vi "Digilens DLP Gen2 UI .vi"(11 "TopLevel In":refnum<class "TopLevel.lvclass">) -> (3 "TopLevel Out":refnum<class "TopLevel.lvclass">)   [LabVIEW 2022 SP3, in "TopLevel.lvclass"] (continued)
    shift-left: _ -> [w28]
    shift-right: [w32] -> _
    shift-left: w6 -> [w26]
    shift-right: [w31] -> _
    shift-left: w16 -> [w33]
    tunnel: w5 -> [w25]
    tunnel: [w24] -> w14
    shift-right: [w23] -> _
    shift-left: _ -> [w22]
    tunnel: w7 -> [_]
    tunnel: w1 -> [w21]
    tunnel: w2 -> [w20]
    stop <- w30 stop-if-true
    w27 = -1  # Timeout
    n10 = call <vilib>:"Parse State Queue__JKI_lib_State_Machine.vi"("State Queue"=w33, "Error In (no error)"=w26) -> ("Remaining States"=w35:string, "Current State"=w36:string, "Arguments"=w34:string)  [unwired: 11 in]
    n11 = case shown="\"Action: Apply Process Mode\"" w36 {
      selector: w36 -> [_ _ w2966 _ _ _ _ _ _ _ _ _ _ _ _ _ _ _ _ _ _ _ _ _ _ _ _ _ _ _ _ _ _ _ _ _ _ _ _ _ _ _ _ _ _ _ _ _ _ _ _ _ _ _ _ _ _ _ _ _ _ _ _ _ _ _ _ _ _ _ _ _ _ _ _ _ _ _ _ _ _ _ _ _ _ _ _ _ _]
      tunnel: w35 -> [w46 w2963 w2970 w2990 w2998 w3005 w3011 w3023 w3036 w3056 w3067 w3078 w3098 w3123 w3140 w3152 w3158 w3206 w3325 w3339 w3351 w3357 w3365 w3373 w3388 w3428 w3519 w3605 w3616 w3626 w3637 w3662 w3706 w3716 w3750 w3756 w3780 w3793 w3891 w3913 w3934 w3947 w3984 w4007 w4014 w4021 w4040 w4045 w4079 w4087 w4092 w4106 w4108 w4119 w4140 w4145 w4154 w4164 w4168 w4181 w4185 w4193 w4238 w4249 w4282 w4309 w4360 w4405 w4409 w4438 w4514 w4521 w4528 w4530 w4567 w4619 w4660 w4689 w4693 w4703 w4707 w4710 w4726 w4730 w4775 w4819 w4824 w4839 w4863]
      tunnel: w34 -> [_ _ _ _ _ _ _ _ _ _ _ _ w3086 w3109 w3130 w3148 _ _ _ _ _ _ w3358 _ _ _ w3513 _ _ _ _ _ _ _ _ _ _ _ _ w3905 w3929 w3942 _ _ _ _ _ _ _ _ _ _ _ _ _ _ _ _ _ _ _ w4190 _ w4248 _ _ _ _ _ w4430 _ _ _ _ _ _ _ _ _ _ _ _ _ w4728 w4768 _ _ w4833 w4859]
      tunnel: w28 -> [w44 w2960 w2968 w2981 w2995 w3003 w3008 w3019 w3034 w3053 w3063 w3072 w3084 w3115 w3129 w3142 w3153 w3202 _ w3338 w3346 w3354 w3362 w3370 w3383 w3441 w3516 w3600 w3612 w3621 w3634 w3658 w3701 w3711 w3745 w3751 w3775 w3790 w3888 w3908 w3932 w3944 w3981 w4004 w4011 w4018 w4028 w4043 w4075 w4086 w4090 w4094 w4112 w4117 w4139 w4144 w4151 w4161 w4167 w4179 w4184 w4189 w4241 w4245 w4278 w4296 w4348 w4399 w4408 w4445 w4511 w4518 w4525 w4557 w4582 w4622 w4657 w4681 w4692 w4700 w4706 w4716 w4725 w4732 w4777 w4818 w4823 w4834 w4860]
      tunnel: [w43 w2961 w2972 w2987 errorcluster {"status"=FALSE, "code"=0, "source"=""} ("error out") w3002 w3009 w3012 w3025 w3054 w3061 w3070 w3088 w3111 w3126 w3144 w3156 w3200 w3265 w3329 w3347 w3355 w3363 w3371 w3386 w3422 w3517 w3603 w3610 w3624 w3635 w3654 w3704 w3714 w3748 w3754 w3778 w3783 w3836 w3911 w3930 w3939 w3977 w4008 w4012 w4019 w4027 w4044 w4058 w4083 w4091 w4093 w4109 w4114 w4141 w4146 w4148 w4159 w4169 w4176 w4186 w4188 w4234 w4251 w4262 w4299 w4350 w4398 w4410 w4441 w4496 w4516 w4522 w4532 w4572 w4615 w4630 w4685 w4694 w4696 w4708 w4715 w4727 w4735 w4780 w4820 w4825 w4835 w4851] -> w32
      tunnel: w26 -> [w42 w2961 w2971 w2987 w2994 w3002 w3009 w3017 w3024 w3054 w3060 w3069 w3087 w3110 w3125 w3143 w3156 w3199 w3307 w3333 w3348 w3355 w3363 w3371 w3386 w3417 w3517 w3603 w3609 w3624 w3635 w3653 w3704 w3714 w3748 w3754 w3778 w3782 w3836 w3911 w3931 w3945 w3971 w4008 w4012 w4019 w4026 w4044 w4048 w4082 w4091 w4096 w4109 w4113 w4141 w4146 w4147 w4158 w4169 w4175 w4186 w4187 w4244 w4253 w4261 w4295 w4347 w4397 w4410 w4440 w4508 w4515 w4523 w4544 w4579 w4621 w4646 w4684 w4694 w4695 w4708 w4714 w4727 w4734 w4779 w4820 w4825 w4828 w4856]
      tunnel: [w45 w2962 w2969 w2989 w2997 w3004 w3010 w3022 w3035 w3055 w3066 w3078 w3097 w3122 w3139 w3151 w3157 w3205 w3324 w3339 w3350 w3356 w3364 w3372 w3387 w3427 w3518 w3604 w3615 w3625 w3636 w3661 w3705 w3715 w3749 w3755 w3779 w3793 w3891 w3912 w3933 w3946 w3984 w4007 w4013 w4020 w4039 w4045 w4079 w4087 w4092 w4106 w4108 w4119 w4140 w4145 w4154 w4164 w4168 w4181 w4185 w4193 w4239 w4250 w4282 w4309 w4360 w4405 w4409 w4439 w4514 w4521 w4528 w4531 w4568 w4620 w4660 w4689 w4693 w4703 w4707 w4711 w4726 w4731 w4776 w4819 w4824 w4839 w4863] -> w31
      tunnel: [_ _ _ _ _ TRUE _ _ _ _ _ _ _ _ _ _ _ _ _ _ _ _ _ _ _ _ _ _ _ _ _ _ _ _ _ _ _ _ _ _ _ _ _ _ _ _ _ _ _ _ _ _ _ _ _ _ _ _ _ _ _ _ _ _ _ _ _ _ _ _ _ _ _ _ _ _ _ _ _ _ _ _ _ _ _ _ _ _ _] -> w30
      tunnel: [w41 w2960 w2968 w2988 w2995 w3003 w3008 w3016 w3034 w3050 w3059 w3072 w3085 w3115 w3129 w3142 w3153 w3198 w3323 w3332 w3346 w3354 w3362 w3370 w3383 w3432 w3516 w3600 w3612 w3621 w3634 w3658 w3701 w3711 w3745 w3751 w3775 w3789 w3888 w3908 w3932 w3944 w3981 w4004 w4011 w4018 w4028 w4043 w4075 w4086 w4090 w4094 w4112 w4117 w4139 w4144 w4151 w4161 w4167 w4179 w4184 w4189 w4241 w4246 w4278 w4296 w4348 w4399 w4408 w4445 w4509 w4518 w4525 w4538 w4582 w4617 w4638 w4681 w4692 w4700 w4706 w4713 w4725 w4733 w4778 w4818 w4823 w4834 w4860] -> w29
      tunnel: w27 -> [w40 _ _ _ _ _ _ _ _ _ _ _ _ _ _ _ _ _ _ _ _ _ _ _ _ _ _ _ _ _ _ _ _ _ _ _ _ _ _ _ _ _ _ _ _ _ _ _ _ _ _ _ _ _ _ _ _ _ _ _ _ _ _ _ _ _ _ _ _ _ _ _ _ _ _ _ _ _ _ _ _ _ _ _ _ _ _ _ _]
      tunnel: w25 -> [w39 w2959 w2965 w2978 w2992 w3000 w3007 w3021 w3033 w3052 w3065 w3077 w3096 w3121 w3138 w3150 w3155 w3204 w3321 w3337 w3345 w3353 w3361 w3369 w3384 w3446 w3515 w3602 w3614 w3623 w3633 w3660 w3703 w3713 w3747 w3753 w3777 w3792 w3890 w3910 w3928 w3941 w3983 w4006 w4010 w4016 w4031 w4042 w4078 w4085 w4089 w4097 w4111 w4121 w4138 w4143 w4153 w4163 w4166 w4177 w4183 w4192 w4243 w4255 w4281 w4308 w4359 w4404 w4407 w4449 w4513 w4520 w4527 w4559 w4591 w4624 w4659 w4686 w4691 w4702 w4705 w4722 w4724 w4743 w4788 w4817 w4822 w4838 w4862]
      tunnel: [w38 w2959 w2965 w2978 w2992 w3000 w3007 w3021 w3033 w3052 w3065 w3077 w3096 w3121 w3138 w3150 w3155 w3204 w3321 w3337 w3345 w3353 w3361 w3369 w3384 w3446 w3515 w3602 w3614 w3623 w3633 w3660 w3703 w3713 w3747 w3753 w3777 w3792 w3890 w3910 w3928 w3941 w3983 w4006 w4010 w4016 w4031 w4042 w4078 w4085 w4089 w4097 w4111 w4121 w4138 w4143 w4153 w4163 w4166 w4178 w4183 w4192 w4243 w4255 w4281 w4308 w4359 w4404 w4407 w4449 w4513 w4520 w4527 w4559 w4591 w4624 w4659 w4687 w4691 w4702 w4705 w4722 w4724 w4743 w4788 w4817 w4822 w4838 w4862] -> w24
      tunnel: [w37 w2958 w2964 w2977 w2991 w2999 w3006 w3020 w3032 w3051 w3064 w3076 w3095 w3120 w3137 w3149 w3154 w3203 w3311 w3336 w3344 w3352 w3360 w3368 w3385 w3445 w3514 w3601 w3613 w3622 w3632 w3659 w3702 w3712 w3746 w3752 w3776 w3791 w3889 w3909 w3927 w3940 w3982 w4005 w4009 w4015 w4032 w4041 w4074 w4084 w4088 w4105 w4110 w4120 w4137 w4142 w4152 w4162 w4165 w4180 w4182 w4191 w4242 w4254 w4280 w4307 w4358 w4403 w4406 w4448 w4512 w4519 w4526 w4558 w4590 w4623 w4658 w4688 w4690 w4701 w4704 w4721 w4723 w4742 w4787 w4816 w4821 w4837 w4861] -> w23
      tunnel: w22 -> [w37 w2958 w2964 w2977 w2991 w2999 w3006 w3020 w3032 w3051 w3064 w3076 w3095 w3120 w3137 w3149 w3154 w3203 w3311 w3336 w3344 w3352 w3360 w3368 w3385 w3445 w3514 w3601 w3613 w3622 w3632 w3659 w3702 w3712 w3746 w3752 w3776 w3791 w3889 w3909 w3927 w3940 w3982 w4005 w4009 w4015 w4032 w4041 _ w4084 w4088 w4105 w4110 w4120 w4137 w4142 w4152 w4162 w4165 w4180 w4182 w4191 w4242 w4254 w4280 w4307 w4358 w4403 w4406 w4448 w4512 w4519 w4526 w4558 w4590 w4623 w4658 w4688 w4690 w4701 w4704 w4721 w4723 w4742 w4787 w4816 w4821 w4837 w4861]
      tunnel: w21 -> [_ _ _ _ _ _ _ _ _ _ _ _ _ _ _ w3145 _ _ _ _ _ _ _ _ _ _ _ _ _ _ _ _ _ _ _ _ _ _ _ _ _ _ _ _ _ _ w4024 _ _ _ _ _ _ _ _ _ _ _ _ _ _ _ _ _ _ _ _ _ _ _ _ _ _ _ _ _ _ _ _ _ _ _ _ _ _ _ _ _ _]
      tunnel: w20 -> [_ _ _ _ _ _ _ _ _ _ _ _ _ _ _ _ _ _ _ _ _ _ _ _ _ w3431 _ _ _ _ _ _ _ _ _ _ _ _ _ _ _ _ _ _ _ _ _ _ _ _ _ _ _ _ _ _ _ _ _ _ _ _ _ _ _ _ _ _ _ _ _ _ _ _ _ _ _ _ _ _ _ _ _ _ _ _ _ _ _]
      frame "", "Event Structure", "Idle" {
        n12 = event shown="[7] \"SaveMeniscusinXML\": Value Change" {
          selector: w37 -> [_ _ _ _ _ _ _ _ _ _ _ _ _ _ _ _ _ _ _ _ _ _ _ _ _ _ _ _ _ _ _ _ _ _ _ _ _ _ _ _ _ _ _ _ _ _ _ w791 _ _ _ _ _ _ _ _ _ _ _ _ _ _ _ _ _ _ _ _ _ _ _ _ _ _ _ _ _ _ _ _ _ _ _ _ _ _ _ _ _ _ _ _ _ _ _ _ _ _ _ _ _ _ _ _ _ _ _ _ _ _ _ _ _ _ _ _ _ _ _ _ _ _ _ _ _ _ _ _ _ _ _ _ _ _ _ _ _ _ _ _ _ _]
          dyn-events: [_ _ _ _ _ _ _ _ _ _ _ _ _ _ _ _ _ _ _ _ _ _ _ _ _ _ _ _ _ _ _ _ _ _ _ _ _ _ _ _ _ _ _ _ _ _ _ w788 _ _ _ _ _ _ _ _ _ _ _ _ _ _ _ _ _ _ _ _ _ _ _ _ _ _ _ _ _ _ _ _ _ _ _ _ _ _ _ _ _ _ _ _ _ _ _ _ _ _ _ _ _ _ _ _ _ _ _ _ _ _ _ _ _ _ _ _ _ _ _ _ _ _ _ _ _ _ _ _ _ _ _ _ _ _ _ _ _ _ _ _ _ _] -> _
          timeout: w40 -> [_ _ _ _ _ _ _ _ _ _ _ _ _ _ _ _ _ _ _ _ _ _ _ _ _ _ _ _ _ _ _ _ _ _ _ _ _ _ _ _ _ _ _ _ _ _ _ _ _ _ _ _ _ _ _ _ _ _ _ _ _ _ _ _ _ _ _ _ _ _ _ _ _ _ _ _ _ _ _ _ _ _ _ _ _ _ _ _ _ _ _ _ _ _ _ _ _ _ _ _ _ _ _ _ _ _ _ _ _ _ _ _ _ _ _ _ _ _ _ _ _ _ _ _ _ _ _ _ _ _ _ _ _ _ _ _ _ _ _ _ _ _]
          tunnel: w46 -> [w51 w57 w69 w77 w94 w106 w112 w118 w127 w136 w160 w167 w179 w186 w196 w206 w216 w228 w237 w245 w255 w271 w319 w356 w368 w391 w421 w444 w457 w478 w484 w490 w496 w507 w516 w534 w621 w666 w674 w688 w694 w703 w721 w736 w743 w754 w757 w792 w813 w830 w843 w859 w886 w895 w904 w913 w922 w931 w959 w980 w1003 w1026 w1049 w1072 w1095 w1121 w1134 w1140 w1174 w1209 w1225 w1232 w1245 w1266 w1282 w1292 w1302 w1320 w1331 w1350 w1369 w1388 w1407 w1426 w1450 w1493 w1537 w1573 w1609 w1645 w1681 w1717 w1754 w1756 w1782 w1798 w1820 w1841 w1862 w1883 w1905 w1926 w1957 w1989 w2022 w2055 w2088 w2121 w2153 w2185 w2217 w2250 w2283 w2315 w2348 w2381 w2414 w2447 w2480 w2513 w2534 w2555 w2576 w2597 w2618 w2665 w2733 w2754 w2775 w2796 w2817 w2838 w2859 w2875 w2893 w2912 w2919 w2926 w2933 w2940 w2947 w2953]
          tunnel: [w50 w56 w68 w76 w93 w105 w111 w117 w126 w135 w159 w166 w178 w185 w195 w205 w215 w227 w236 w244 w254 w270 w318 w355 w367 w390 w422 w443 w456 w477 w483 w489 w495 w506 w515 w533 w620 w665 w673 w687 w693 w702 w720 w735 w742 w753 w758 w793 w813 w830 w843 w859 w887 w896 w905 w914 w923 w932 w958 w981 w1004 w1027 w1050 w1073 w1096 w1121 w1134 w1140 w1174 w1209 w1225 w1232 w1245 w1266 w1282 w1292 w1302 w1320 w1332 w1351 w1370 w1389 w1408 w1427 w1451 w1493 w1537 w1573 w1609 w1645 w1681 w1717 w1754 w1757 w1783 w1798 w1820 w1841 w1862 w1883 w1905 w1926 w1957 w1989 w2022 w2055 w2088 w2121 w2153 w2185 w2217 w2250 w2283 w2315 w2348 w2381 w2414 w2447 w2480 w2513 w2534 w2555 w2576 w2597 w2618 w2665 w2733 w2754 w2775 w2796 w2817 w2838 w2859 w2876 w2892 w2911 w2918 w2925 w2932 w2939 w2946 w2954] -> w45
          tunnel: w44 -> [w48 w54 w63 w71 w91 w101 w109 w115 w124 w132 w157 w164 w176 w183 w193 w203 w211 w224 w235 w242 w252 w268 w297 w327 w365 w388 w424 w441 w454 w475 w481 w487 w493 w502 w513 w525 w611 w663 w672 w685 w691 w700 w718 w733 w738 w751 w775 w795 w801 w829 w842 w853 w891 w900 w909 w918 w927 w936 w963 w982 w1005 w1028 w1051 w1074 w1097 w1118 w1128 w1137 w1169 w1207 w1223 w1230 w1243 w1264 w1280 w1290 w1300 w1314 w1327 w1341 w1361 w1380 w1399 w1418 w1445 w1488 w1534 w1568 w1604 w1640 w1676 w1712 w1742 w1759 w1788 w1796 w1817 w1838 w1859 w1880 w1902 w1923 w1954 w1986 w2019 w2052 w2085 w2118 w2150 w2182 w2214 w2247 w2280 w2312 w2345 w2378 w2411 w2444 w2477 w2510 w2531 w2552 w2573 w2594 w2615 w2662 w2731 w2751 w2772 w2793 w2814 w2835 w2856 w2878 w2895 w2914 w2921 w2928 w2935 w2942 w2949 w2956]
          tunnel: [w49 w55 w59 w75 w88 w104 w110 w116 w125 w130 w158 w165 w177 w184 w194 w204 w214 w226 w231 w243 w253 w258 w317 w323 w357 w384 w425 w442 w455 w476 w482 w488 w494 w498 w514 w518 w619 w664 w669 w678 w692 w701 w711 w729 w737 w750 w776 w787 w797 w827 w840 w852 w892 w901 w910 w919 w928 w937 w961 w977 w1000 w1023 w1046 w1069 w1092 w1117 w1127 w1136 w1141 w1197 w1211 w1227 w1234 w1254 w1268 w1288 w1298 w1307 w1334 w1353 w1372 w1391 w1410 w1429 w1435 w1473 w1535 w1570 w1606 w1642 w1678 w1714 w1751 w1766 w1786 w1793 w1815 w1836 w1857 w1878 w1900 w1921 w1952 w1984 w2017 w2050 w2083 w2116 w2148 w2180 w2212 w2245 w2278 w2310 w2343 w2376 w2409 w2442 w2475 w2508 w2529 w2550 w2571 w2592 w2613 w2649 w2728 w2749 w2770 w2791 w2812 w2833 w2854 w2877 w2889 w2915 w2922 w2929 w2936 w2943 w2950 w2952] -> w43
          tunnel: w42 -> [w49 w55 w58 w75 w88 w104 w110 w116 w125 w129 w158 w165 w177 w184 w194 w204 w214 w226 w230 w243 w253 w266 w317 w324 w363 w386 w425 w442 w455 w476 w482 w488 w494 w497 w514 w517 w619 w664 w668 w683 w692 w701 w705 w728 w737 w750 w776 w786 w811 w826 w839 w851 w892 w901 w910 w919 w928 w937 w960 w976 w999 w1022 w1045 w1068 w1091 w1116 w1126 w1135 w1156 w1191 w1215 w1228 w1235 w1247 w1272 w1287 w1297 w1313 w1334 w1353 w1372 w1391 w1410 w1429 w1436 w1490 w1530 w1571 w1607 w1643 w1679 w1715 w1750 w1765 w1785 w1792 w1814 w1835 w1856 w1877 w1899 w1920 w1951 w1983 w2016 w2049 w2082 w2115 w2147 w2179 w2211 w2244 w2277 w2309 w2342 w2375 w2408 w2441 w2474 w2507 w2528 w2549 w2570 w2591 w2612 w2640 w2727 w2748 w2769 w2790 w2811 w2832 w2853 w2877 w2888 w2915 w2922 w2929 w2936 w2943 w2950 w2952]
          tunnel: [w48 w54 w63 w72 w86 w102 w109 w115 w122 w132 w157 w164 w176 w183 w193 w203 w211 w224 w235 w242 w252 w268 w295 w347 w365 w388 w424 w441 w454 w475 w481 w487 w493 w502 w513 w523 w612 w661 w672 w677 w691 w700 w718 w733 w738 w751 w764 w795 w801 w829 w842 w853 w889 w898 w907 w916 w925 w934 w963 w983 w1006 w1029 w1052 w1075 w1098 w1118 w1128 w1137 w1169 w1207 w1223 w1230 w1243 w1264 w1280 w1290 w1300 w1314 w1333 w1352 w1371 w1390 w1409 w1428 w1448 w1488 w1533 w1569 w1605 w1641 w1677 w1713 w1742 w1759 w1788 w1796 w1817 w1838 w1859 w1880 w1902 w1923 w1954 w1986 w2019 w2052 w2085 w2118 w2150 w2182 w2214 w2247 w2280 w2312 w2345 w2378 w2411 w2444 w2477 w2510 w2531 w2552 w2573 w2594 w2615 w2662 w2731 w2751 w2772 w2793 w2814 w2835 w2856 w2878 w2895 w2914 w2921 w2928 w2935 w2942 w2949 w2956] -> w41
          tunnel: w39 -> [w47 w53 w67 w74 w92 w103 w108 w114 w123 w133 w156 w163 w175 w182 w192 w202 w213 w225 w234 w241 w251 w269 w316 w354 w366 w389 w423 w440 w453 w474 w480 w486 w492 w505 w512 w532 w618 w662 w670 w686 w690 w699 w719 w734 w739 w752 w774 w794 w814 w831 w844 w858 w890 w899 w908 w917 w926 w935 w962 w978 w1001 w1024 w1047 w1070 w1093 w1120 w1133 w1139 w1173 w1208 w1224 w1231 w1244 w1265 w1281 w1291 w1301 w1319 w1335 w1354 w1373 w1392 w1411 w1430 w1452 w1492 w1536 w1572 w1608 w1644 w1680 w1716 w1752 w1767 w1789 w1797 w1818 w1839 w1860 w1881 w1903 w1924 w1955 w1987 w2020 w2053 w2086 w2119 w2151 w2183 w2215 w2248 w2281 w2313 w2346 w2379 w2412 w2445 w2478 w2511 w2532 w2553 w2574 w2595 w2616 w2663 w2732 w2752 w2773 w2794 w2815 w2836 w2857 w2879 w2894 w2913 w2920 w2927 w2934 w2941 w2948 w2957]
          tunnel: [w47 w53 w67 w74 w92 w103 w108 w114 w123 w133 w156 w163 w175 w182 w192 w202 w213 w225 w234 w241 w251 w269 w316 w354 w366 w389 w423 w440 w453 w474 w480 w486 w492 w505 w512 w532 w618 w662 w671 w686 w690 w699 w719 w734 w739 w752 w774 w794 w814 w831 w844 w858 w890 w899 w908 w917 w926 w935 w962 w978 w1001 w1024 w1047 w1070 w1093 w1120 w1133 w1139 w1173 w1208 w1224 w1231 w1244 w1265 w1281 w1291 w1301 w1319 w1335 w1354 w1373 w1392 w1411 w1430 w1452 w1492 w1536 w1572 w1608 w1644 w1680 w1716 w1753 w1768 w1789 w1797 w1818 w1839 w1860 w1881 w1903 w1924 w1955 w1987 w2020 w2053 w2086 w2119 w2151 w2183 w2215 w2248 w2281 w2313 w2346 w2379 w2412 w2445 w2478 w2511 w2532 w2553 w2574 w2595 w2616 w2663 w2732 w2752 w2773 w2794 w2815 w2836 w2857 w2879 w2894 w2913 w2920 w2927 w2934 w2941 w2948 w2957] -> w38
          event Timeout {
            n13 = event-data() -> ()  [unwired: 1 in, 1 out]
            n14 = call <vilib>:"Add State(s) to Queue__JKI_lib_State_Machine.vi"("State(s) in (\"\")"=w51) -> ("States Out"=w50:string)  [unwired: 14 in]
          }
          event "PrintHead Number": Value Change {
            n15 = event-data() -> ()  [unwired: 1 in, 6 out]
            n16 = call <vilib>:"Add State(s) to Queue__JKI_lib_State_Machine.vi"("State(s) in Front (\"\")"="Action: LoadImages>>CalibrationPrints" ("State(s) in Front (\"\")"), "State(s) in (\"\")"=w57) -> ("States Out"=w56:string)  [unwired: 13 in]
          }
          event "Refresh Timer": Value Change {
            n17 = event-data() -> ()  [unwired: 1 in, 6 out]
            n18 = Unbundle By Name(w63) -> ("TopLevel out"=w62:refnum<class "TopLevel.lvclass">, "DAQ"=w61:refnum<class "DAQ.lvclass">)
            n19 = call "Generate Timer Event.vi"("error in (no error)"=w58, "CmdMsg"="Init", "DAQ"=w61) -> ("error out"=w60:errorcluster)  [unwired: 7 in, 1 out]
            n20 = call-dynamic "Generate PurgeRequestEvent.vi"("error in (no error)"=w60, "Command"="TimerElapsed" ("CmdMsg"), "TopLevel in"=w62) -> ("error out"=w59:errorcluster)  [unwired: 7 in, 1 out]
            n21 = call <vilib>:"Add State(s) to Queue__JKI_lib_State_Machine.vi"("State(s) in Front (\"\")"="" ("State(s) in Front (\"\")"), "State(s) in (\"\")"=w69) -> ("States Out"=w68:string)  [unwired: 13 in]
          }
          event User Event {
            n22 = event-data() -> ("Command"=w73:string)  [unwired: 1 in, 5 out]
            n23 = case shown="\"Done\"" w73 {
              tunnel: w71 -> [w78 w80 w84]
              tunnel: [w78 w80 w83] -> w72
              tunnel: [_ "UI: EnableControls>>Print PPP Image>>False\nUI: EnableControls>>PrimeHeads>>True" "UI: EnableControls>>Print PPP Image>>True\nUI: EnableControls>>PrimeHeads>>False\nAction: PrePrimeTimer>>Enable"] -> w70
              frame Default {
              }
              frame "TimerElapsed" {
              }
              frame "Done" {
                n24 = Bundle By Name(cluster=w84, "PrePrimeDone"=TRUE) -> (w83:T77)
              }
            }
            n25 = call <vilib>:"Add State(s) to Queue__JKI_lib_State_Machine.vi"("State(s) in Front (\"\")"=w70, "State(s) in (\"\")"=w77) -> ("States Out"=w76:string)  [unwired: 13 in]
          }
          event "EnableHeadPrimeTimer": Value Change {
            # "timer not enabled. alway show button to print"
            n26 = event-data() -> ("NewVal"=w85:bool)  [unwired: 1 in, 5 out]
            n27 = Select(t="Action: PrePrimeTimer>>Enable\nUI: EnableControls>>Print PPP Image>>False\nUI: EnableControls>>PrimeHeads>>True", s=w85, f="Action: PrePrimeTimer>>Disable\nUI: EnableControls>>Print PPP Image>>True\nUI: EnableControls>>PrimeHeads>>False") -> (s? t:f=w87:string)
            n28 = Bundle By Name(cluster=w91, "PrePrimeTmrEnabled"=w85) -> (w86:T77)
            n29 = call <vilib>:"Add State(s) to Queue__JKI_lib_State_Machine.vi"("State(s) in Front (\"\")"=w87, "State(s) in (\"\")"=w94) -> ("States Out"=w93:string)  [unwired: 13 in]
          }
          event "Weights 1", "Weights 2", "Weights 3", "Weights 4", "Weights 5", "Weights 6": Value Change {
            n30 = event-data() -> ()  [unwired: 1 in, 6 out]
            n31 = Bundle By Name(cluster=w101, "PrintWeights.Weights 1"="Weights 1", "PrintWeights.Weights 2"="Weights 2", "PrintWeights.Weights 3"="Weights 3", "PrintWeights.Weights 4"="Weights 4", "PrintWeights.Weights 5"="Weights 5", "PrintWeights.Weights 6"="Weights 6") -> (w102:T77)
            n32 = call <vilib>:"Add State(s) to Queue__JKI_lib_State_Machine.vi"("State(s) in (\"\")"=w106) -> ("States Out"=w105:string)  [unwired: 14 in]
          }
          event "SaveINIXML": Value Change {
            n33 = event-data() -> ()  [unwired: 1 in, 6 out]
            n34 = call <vilib>:"Add State(s) to Queue__JKI_lib_State_Machine.vi"("State(s) in Front (\"\")"="Action: Update Materials in XML\nAction: Update PrintWeights in XML\nAction: Update INI XML" ("State(s) in Front (\"\")"), "State(s) in (\"\")"=w112) -> ("States Out"=w111:string)  [unwired: 13 in]
          }
          event "SaveMeniscusinXML": Value Change {
            n35 = event-data() -> ()  [unwired: 1 in, 6 out]
            n36 = call <vilib>:"Add State(s) to Queue__JKI_lib_State_Machine.vi"("State(s) in Front (\"\")"="Action: Update MeniscusPressure in XML\nAction: Update INI XML" ("State(s) in Front (\"\")"), "State(s) in (\"\")"=w118) -> ("States Out"=w117:string)  [unwired: 13 in]
          }
          event User Event {
            n37 = event-data() -> ("UserLevel"=w121:T76, "Login Time"=w120:timestamp)  [unwired: 1 in, 4 out]
            n38 = Bundle By Name(cluster=w124, "Login.UserLevel"=w121, "Login.Login Time"=w120) -> (w122:T77)
            n39 = call <vilib>:"Add State(s) to Queue__JKI_lib_State_Machine.vi"("State(s) in Front (\"\")"="UI: Process Login Event" ("State(s) in Front (\"\")"), "State(s) in (\"\")"=w127) -> ("States Out"=w126:string)  [unwired: 13 in]
          }
          event "Login": Value Change {
            n40 = event-data() -> ("NewVal"=w134:bool)  [unwired: 1 in, 5 out]
            n41 = Unbundle By Name(w132) -> ("TopLevel out"=w131:refnum<class "TopLevel.lvclass">)
            n42 = case shown="True" w134 {
              tunnel: w131 -> [w138 w150]
              tunnel: w129 -> [w140 w149]
              tunnel: [w139 w148] -> w130
              tunnel: [w137 _] -> w128
              frame False {
                n43 = call <vilib>:"Three Button Dialog.vi"("Center Button Text (\"No\")"="" ("Center Button Text (\"No\")"), "message"="Are you sure you want to Logout?") -> ("Which Button?"=w141:T78)  [unwired: 9 in]
                n44 = case shown="\"Left Button\"" w141 {
                  tunnel: w140 -> [w144 w146 w147]
                  tunnel: [w144 w146 w147] -> w139
                  tunnel: w138 -> [_ _ _]
                  tunnel: ["UI: Request Logout" ("State(s) in Front (\"\")") _ _] -> w137
                  frame "Left Button" {
                  }
                  frame "Center Button", Default {
                  }
                  frame "Right Button" {
                  }
                }
              }
              frame True {
                n45 = call "SendLogInRequestEvent.vi"("error in (no error)"=w149, "TopLevel in"=w150) -> ("error out"=w148:errorcluster)  [unwired: 8 in, 1 out]
              }
            }
            n46 = call <vilib>:"Add State(s) to Queue__JKI_lib_State_Machine.vi"("State(s) in Front (\"\")"=w128, "State(s) in (\"\")"=w136) -> ("States Out"=w135:string)  [unwired: 13 in]
          }
          event "Load Calibration Rx": Value Change {
            n47 = event-data() -> ()  [unwired: 1 in, 6 out]
            n48 = property on="Recipe" class="Ring (strict)"() -> ("RingText.Text"=w155:string)  [unwired: 2 in, 2 out]
            n49 = Concatenate Strings("Data: LoadRecipe>>" ("string"), w155) -> (w154:string)
            n50 = Format Into String(format string="%s\nUI: Update Calibration Heads\nAction: LoadImages>>CalibrationPrints", w154) -> (resulting string=w151:string)  [unwired: 2 in, 1 out]
            n51 = call <vilib>:"Add State(s) to Queue__JKI_lib_State_Machine.vi"("State(s) in Front (\"\")"=w151, "State(s) in (\"\")"=w160) -> ("States Out"=w159:string)  [unwired: 13 in]
          }
          event "Recipe": Value Change {
            n52 = event-data() -> ()  [unwired: 1 in, 6 out]
            n53 = property on="RecipeType" class="Ring (strict)"() -> ("RingText.Text"=w161:string)  [unwired: 2 in, 2 out]
            n54 = case shown="\"Calibration\"" w161 {
              selector: w161 -> [w172 _ _]
              frame Default {
                w169 = "\r"
                n55 = Concatenate Strings("Unsupported Recipe Type: " ("string"), w172, w169, "Recipe Type can only be of type \"Calibration\" or \"PrintDesign\"" ("string"), w169, "Please contact Engineer" ("string")) -> (w171:string)
                n56 = One Button Dialog(message=w171) -> ()  [unwired: 1 in, 1 out]
              }
              frame "Calibration" {
              }
              frame "PrintDesign" {
              }
            }
            n57 = call <vilib>:"Add State(s) to Queue__JKI_lib_State_Machine.vi"("State(s) in Front (\"\")"="UI: EnableControls>>RIP Recipe>>True\nUI: EnableControls>>Load Calibration Rx>>True\nUI: EnableControls>>Print PPP Image>>False\nUI: EnableControls>>Head Print Command>>False" ("State(s) in Front (\"\")"), "State(s) in (\"\")"=w167) -> ("States Out"=w166:string)  [unwired: 13 in]
          }
          event "Refresh": Value Change {
            n58 = event-data() -> ()  [unwired: 1 in, 6 out]
            n59 = call <vilib>:"Add State(s) to Queue__JKI_lib_State_Machine.vi"("State(s) in Front (\"\")"="Action: Sort Recipes\nUI: Update Status>>Refresh Recipe List\nUI: Init Recipe Dropdowns\nUI: EnableControls>>Load Customer Design>>True\nUI: EnableControls>>RIP Recipe>>True\nUI: EnableControls>>Print PPP Image>>False\nUI: EnableControls>>Head Print Command>>False" ("State(s) in Front (\"\")"), "State(s) in (\"\")"=w179) -> ("States Out"=w178:string)  [unwired: 13 in]
          }
          event "ImageMain 2", "ImageMain 4", "ImageMain 3", "ImageMain 5": Shortcut Menu Selection (User) {
            n60 = event-data() -> ("CtlRef"=w181:refnum<vi>)  [unwired: 1 in, 7 out]
            n61 = property class="ImageControl"(reference=w181, "Zoom to Fit Mode"=TRUE) -> ()  [unwired: 1 in, 2 out]
            n62 = call <vilib>:"Add State(s) to Queue__JKI_lib_State_Machine.vi"("State(s) in (\"\")"=w186) -> ("States Out"=w185:string)  [unwired: 14 in]
          }
          event "StartPrintSequence": Value Change {
            n63 = event-data() -> ()  [unwired: 1 in, 6 out]
            n64 = property on="Recipe" class="Ring (strict)"() -> ("RingText.Text"=w191:string)  [unwired: 2 in, 2 out]
            n65 = Concatenate Strings("Data: LoadRecipe>>" ("string"), w191) -> (w190:string)
            n66 = Format Into String(format string="%s\nUI: Verify and Apply Recipe Details\nAction: Separate Layers\nAction: Invoke PPP\nAction: Print PPP Image", w190) -> (resulting string=w187:string)  [unwired: 2 in, 1 out]
            n67 = call <vilib>:"Add State(s) to Queue__JKI_lib_State_Machine.vi"("State(s) in Front (\"\")"=w187, "State(s) in (\"\")"=w196) -> ("States Out"=w195:string)  [unwired: 13 in]
          }
          event "RIP Recipe": Value Change {
            n68 = event-data() -> ()  [unwired: 1 in, 6 out]
            n69 = property on="Recipe" class="Ring (strict)"() -> ("RingText.Text"=w201:string)  [unwired: 2 in, 2 out]
            n70 = Concatenate Strings("Data: LoadRecipe>>" ("string"), w201) -> (w200:string)
            n71 = Format Into String(format string="%s\nUI: Verify and Apply Recipe Details\nUI: Update Status>>Running Separate Layers\nAction: Separate Layers\nUI: Update Status>>Running PPP\nAction: Invoke PPP", w200) -> (resulting string=w197:string)  [unwired: 2 in, 1 out]
            n72 = call <vilib>:"Add State(s) to Queue__JKI_lib_State_Machine.vi"("State(s) in Front (\"\")"=w197, "State(s) in (\"\")"=w206) -> ("States Out"=w205:string)  [unwired: 13 in]
          }
          event "Print PPP Image": Value Change {
            # "UI: EnableControls>>Print PPP Image>>True"
            n73 = event-data() -> ()  [unwired: 1 in, 6 out]
            n74 = Unbundle By Name(w211) -> ("PrePrimeTmrEnabled"=w210:bool, "PrintDesign.Path"=w208:path)
            n75 = local write "Print PPP Image"(FALSE ("Print PPP Image")) -> ()
            n76 = Empty String/Path?(string/path=w208) -> (empty?=w207:bool)
            n77 = case shown="False" w207 {
              tunnel: w210 -> [w220 _]
              tunnel: [w217 "" ("State(s) in Front (\"\")")] -> w209
              frame False {
                n78 = Select(t="UI: Update Status>>Running PPP Image Print\nAction: Print PPP Image\n/*Action: PrePrimeTimer>>Enable" ("State(s) in Front (\"\")"), s=w220, f="UI: Update Status>>Running PPP Image Print\nAction: Print PPP Image\n/*Action: PrePrimeTimer>>Enable" ("State(s) in Front (\"\")")) -> (s? t:f=w217:string)
              }
              frame True {
                n79 = One Button Dialog(message="Unable to Print. Recipe not Loaded") -> ()  [unwired: 1 in, 1 out]
              }
            }
            n80 = call <vilib>:"Add State(s) to Queue__JKI_lib_State_Machine.vi"("State(s) in Front (\"\")"=w209, "State(s) in (\"\")"=w216) -> ("States Out"=w215:string)  [unwired: 13 in]
          }
          event "PrimeHeads": Value Change {
            # "UI: EnableControls>>Print PPP Image>>True"
            n81 = event-data() -> ()  [unwired: 1 in, 6 out]
            n82 = call <vilib>:"Add State(s) to Queue__JKI_lib_State_Machine.vi"("State(s) in Front (\"\")"="Action: PrePrimeTimer>>Check" ("State(s) in Front (\"\")"), "State(s) in (\"\")"=w228) -> ("States Out"=w227:string)  [unwired: 13 in]
          }
          event Value Change {
            n83 = event-data() -> ("NewVal"=w232:T9)  [unwired: 1 in, 5 out]
            n84 = Format Into String(format string="Action: Apply Process Mode>>%s" ("State(s) in Front (\"\")"), error in=w230, w232) -> (resulting string=w233:string, error out=w231:errorcluster)  [unwired: 1 in]
            n85 = call <vilib>:"Add State(s) to Queue__JKI_lib_State_Machine.vi"("State(s) in Front (\"\")"=w233, "State(s) in (\"\")"=w237) -> ("States Out"=w236:string)  [unwired: 13 in]
          }
          event "Product": Value Change {
            n86 = event-data() -> ()  [unwired: 1 in, 6 out]
            n87 = property on="Product" class="Ring (strict)"() -> ("RingText.Text"=w239:string)  [unwired: 2 in, 2 out]
            n88 = Concatenate Strings("Data: GetProductRecipeNames>>" ("string"), w239) -> (w238:string)
            n89 = call <vilib>:"Add State(s) to Queue__JKI_lib_State_Machine.vi"("State(s) in Front (\"\")"=w238, "State(s) in (\"\")"=w245) -> ("States Out"=w244:string)  [unwired: 13 in]
          }
          event "RecipeType": Value Change {
            n90 = event-data() -> ()  [unwired: 1 in, 6 out]
            n91 = property on="RecipeType" class="Ring (strict)"() -> ("RingText.Text"=w249:string)  [unwired: 2 in, 2 out]
            n92 = case shown="0, Default" "RecipeType" {
              tunnel: [enum32{"Product", "Calibration"}."Product" ("PrintControlTab") enum32{"Product", "Calibration"}."Calibration" ("PrintControlTab")] -> w247
              frame 0, Default {
              }
              frame 1 {
              }
            }
            n93 = property on="PrintControlTab" class="TabCtl (strict)"("Value"=w247) -> ()  [unwired: 2 in, 2 out]
            n94 = Concatenate Strings("Data: Populate Products>>" ("string"), w249) -> (w248:string)
            n95 = call <vilib>:"Add State(s) to Queue__JKI_lib_State_Machine.vi"("State(s) in Front (\"\")"=w248, "State(s) in (\"\")"=w255) -> ("States Out"=w254:string)  [unwired: 13 in]
          }
          event User Event {
            n96 = event-data() -> ()  [unwired: 1 in, 5 out]
            n97 = Unbundle By Name(w268) -> ("DLP2"=w267:refnum<class "DLP2.lvclass">)
            n98 = call "Get SeperatedLayers.vi"("error in (no error)"=w266, "DLP2 in"=w267) -> ("error out"=w259:errorcluster, "Images"=w260:T6[])  [unwired: 7 in, 1 out]
            n99 = for {
              tunnel: w260 -> [w285] mode=indexing
              shift-right: [w281] -> w258
              shift-left: w259 -> [w284]
              tunnel: [w280] -> w265 mode=indexing
              w286 = u32 1 items=["Horizontal", "Vertical", "Central", "1st Diagonal", "2nd Diagonal"] ("Type of Symmetry")
              n100 = call "IMAQ ImageToArray"("error in (no error)"=w284, "Image"=w285) -> ("error out"=w283:errorcluster, "Image Pixels (U8)"=w289:u8[][])  [unwired: 2 in, 3 out]
              n101 = Transpose 2D Array(2D array=w289) -> (transposed array=w288:u8[][])
              n102 = call "IMAQ ArrayToImage"("error in (no error)"=w283, "Image Pixels (U8)"=w288, "Image"=w285) -> ("error out"=w282:errorcluster, "Image Out"=w287:T6)  [unwired: 7 in]
              n103 = call "IMAQ Symmetry"("error in (no error)"=w282, "Type of Symmetry"=w286, "Image Src"=w287) -> ("error out"=w281:errorcluster, "Image Dst Out"=w280:T6)  [unwired: 2 in]
            }
            n104 = Index Array(array=w265) -> (element #1=w261:T6, element #2=w262:T6, element #3=w263:T6, element #4=w264:T6)  [unwired: 4 in]
            n105 = flat-sequence {
              tunnel: w264 -> [w275]
              tunnel: w263 -> [w274]
              tunnel: w262 -> [w273]
              tunnel: w261 -> [w272]
              tunnel: [w279] -> _
              tunnel: [w278] -> _
              tunnel: [w277] -> _
              tunnel: [w276] -> _
              frame #0 {
                "ImageMain 2" <- w272
                "ImageMain 4" <- w273
                "ImageMain 3" <- w274
                "ImageMain 5" <- w275
              }
              frame #1 {
                n106 = invoke on="ImageMain 2" class="ImageControl" method="Refresh Image"() -> (error out=w279:errorcluster)  [unwired: 3 in, 2 out]
                n107 = invoke on="ImageMain 4" class="ImageControl" method="Refresh Image"() -> (error out=w278:errorcluster)  [unwired: 3 in, 2 out]
                n108 = invoke on="ImageMain 3" class="ImageControl" method="Refresh Image"() -> (error out=w277:errorcluster)  [unwired: 3 in, 2 out]
                n109 = invoke on="ImageMain 5" class="ImageControl" method="Refresh Image"() -> (error out=w276:errorcluster)  [unwired: 3 in, 2 out]
              }
            }
            n110 = call <vilib>:"Add State(s) to Queue__JKI_lib_State_Machine.vi"("State(s) in (\"\")"=w271) -> ("States Out"=w270:string)  [unwired: 14 in]
          }
          event User Event {
            n111 = event-data() -> ("PH1_Enable"=w303:bool, "PH2_Enable"=w302:bool, "PH3_Enable"=w301:bool, "PH4_Enable"=w300:bool, "PH5_Enable"=w299:bool, "PH6_Enable"=w298:bool)  [unwired: 1 in, 4 out]
            "H1 Status" <- w303
            "H4 Status" <- w300
            "H5 Status" <- w299
            "H3 Status" <- w301
            "H6 Status" <- w298
            "H2 Status" <- w302
            n112 = Unbundle By Name(w297) -> ("PersistentData.InkChEnable.Enable Ink Ch-1"=w315:bool, "PersistentData.InkChEnable.Enable Ink Ch-2"=w313:bool, "PersistentData.InkChEnable.Enable Ink Ch-3"=w312:bool, "PersistentData.InkChEnable.Enable Ink Ch-4"=w311:bool, "PersistentData.InkChEnable.Enable Ink Ch-5"=w310:bool, "PersistentData.InkChEnable.Enable Ink Ch-6"=w305:bool)
            n113 = Or(x=w303, y=w315) -> (x .or. y?=w314:bool)
            n114 = Or(x=w302, y=w313) -> (x .or. y?=w309:bool)
            n115 = Or(x=w301, y=w312) -> (x .or. y?=w308:bool)
            n116 = Or(x=w300, y=w311) -> (x .or. y?=w307:bool)
            n117 = Or(x=w299, y=w310) -> (x .or. y?=w306:bool)
            n118 = Or(x=w298, y=w305) -> (x .or. y?=w304:bool)
            n119 = Bundle By Name(cluster=w297, "HeadStatusPollData.PH1_Enable"=w303, "HeadStatusPollData.PH2_Enable"=w302, "HeadStatusPollData.PH3_Enable"=w301, "HeadStatusPollData.PH4_Enable"=w300, "HeadStatusPollData.PH5_Enable"=w299, "HeadStatusPollData.PH6_Enable"=w298, "HeadStatus.PH1_Enable"=w314, "HeadStatus.PH2_Enable"=w309, "HeadStatus.PH3_Enable"=w308, "HeadStatus.PH4_Enable"=w307, "HeadStatus.PH5_Enable"=w306, "HeadStatus.PH6_Enable"=w304) -> (w295:T77)
            n120 = Unbundle By Name(w297) -> ("HeadStatus"=w296:T71)
            n121 = Unbundle By Name(w295) -> ("HeadStatus"=w294:T71)
            n122 = Not Equal?(x=w296, y=w294) -> (x != y?=w293:bool)
            n123 = Select(t="UI: Update GIS Controls" ("State(s) in Front (\"\")"), s=w293, f="") -> (s? t:f=w290:string)
            n124 = call <vilib>:"Add State(s) to Queue__JKI_lib_State_Machine.vi"("State(s) in Front (\"\")"=w290, "State(s) in (\"\")"=w319) -> ("States Out"=w318:string)  [unwired: 13 in]
          }
          event User Event {
            # "UI: Update GIS Controls"
            n125 = event-data() -> ("GISHeadStatus"=w325:T70[])  [unwired: 1 in, 4 out]
            n126 = Unbundle By Name(w327) -> ("GISHeadStatus"=w326:T70[])
            n127 = call "EnabledStatusChanged.vi"("error in (no error)"=w324, "GISHeadStatus"=w325, "GISHeadStatus Old"=w326) -> ("error out"=w323:errorcluster, "State"=w321:string)  [unwired: 7 in]
            n128 = Index Array(array=w325) -> (element #1=w353:T70, element #2=w352:T70, element #3=w351:T70, element #4=w350:T70, element #5=w349:T70, element #6=w348:T70)  [unwired: 6 in]
            n129 = Unbundle By Name(w353) -> ("CurrentTemperature"=w346:dbl, "TargetTemperature"=w339:dbl, "HeaterEnabled"=→"HH1 Status":bool)
            "Head 1 Act Temp" <- w346
            n130 = Unbundle By Name(w352) -> ("CurrentTemperature"=w345:dbl, "TargetTemperature"=w338:dbl, "HeaterEnabled"=→"HH2 Status":bool)
            "Head 2 Act Temp" <- w345
            n131 = Unbundle By Name(w349) -> ("CurrentTemperature"=w342:dbl, "TargetTemperature"=w335:dbl, "HeaterEnabled"=→"HH5 Status":bool)
            "Head 5 Act Temp" <- w342
            n132 = Unbundle By Name(w351) -> ("CurrentTemperature"=w344:dbl, "TargetTemperature"=w337:dbl, "HeaterEnabled"=→"HH3 Status":bool)
            "Head 3 Act Temp" <- w344
            n133 = Unbundle By Name(w348) -> ("CurrentTemperature"=w341:dbl, "TargetTemperature"=w334:dbl, "HeaterEnabled"=→"HH6 Status":bool)
            "Head 6 Act Temp" <- w341
            n134 = Unbundle By Name(w350) -> ("CurrentTemperature"=w343:dbl, "TargetTemperature"=w336:dbl, "HeaterEnabled"=→"HH4 Status":bool)
            "Head 4 Act Temp" <- w343
            n135 = Concatenate Strings("UI: Display Heater Temperature", "\n", w321) -> (w322:string)
            n136 = Bundle By Name(cluster=w327, "GISHeadStatus"=w325, "Head Temp.Head 1.Actual"=w346, "Head Temp.Head 1.Target"=w339, "Head Temp.Head 1.Actual"=w345, "Head Temp.Head 1.Target"=w338, "Head Temp.Head 1.Actual"=w344, "Head Temp.Head 1.Target"=w337, "Head Temp.Head 1.Actual"=w343, "Head Temp.Head 1.Target"=w336, "Head Temp.Head 1.Actual"=w342, "Head Temp.Head 1.Target"=w335, "Head Temp.Head 1.Actual"=w341, "Head Temp.Head 1.Target"=w334) -> (w347:T77)
            n137 = call <vilib>:"Add State(s) to Queue__JKI_lib_State_Machine.vi"("State(s) in Front (\"\")"=w322, "State(s) in (\"\")"=w356) -> ("States Out"=w355:string)  [unwired: 13 in]
          }
          event "Head 1 Set", "Head 2 Set", "Head 3 Set", "Head 4 Set", "Head 5 Set", "Head 6 Set": Value Change {
            n138 = event-data() -> ("CtlRef"=w364:refnum<vi>)  [unwired: 1 in, 5 out]
            n139 = property class="Bool"(reference=w364, error in=w363) -> (error out=w357:errorcluster, "Label.Text"=w361:string)  [unwired: 1 out]
            n140 = case shown="\"Head 1 Set\"" w361 {
              tunnel: [0.0 ("Head6 TempSet") "Head1 TempSet" "Head2 TempSet" "Head3 TempSet" "Head4 TempSet" "Head5 TempSet" "Head6 TempSet"] -> w359
              tunnel: [PrinterHeads--Enum."-1" ("Head") PrinterHeads--Enum."1" ("Head") PrinterHeads--Enum."2" ("Head") PrinterHeads--Enum."3" ("Head") PrinterHeads--Enum."4" ("Head") PrinterHeads--Enum."5" ("Head") PrinterHeads--Enum."6" ("Head")] -> w360
              frame Default {
              }
              frame "Head 1 Set" {
              }
              frame "Head 2 Set" {
              }
              frame "Head 3 Set" {
              }
              frame "Head 4 Set" {
              }
              frame "Head 5 Set" {
              }
              frame "Head 6 Set" {
              }
            }
            n141 = Format Into String(format string="Set Head Temperature>>%d>>%f", w360, w359) -> (resulting string=w362:string)  [unwired: 2 in, 1 out]
            n142 = call <vilib>:"Add State(s) to Queue__JKI_lib_State_Machine.vi"("State(s) in Front (\"\")"=w362, "State(s) in (\"\")"=w368) -> ("States Out"=w367:string)  [unwired: 13 in]
          }
          event "Head1 TempSet", "Head2 TempSet", "Head3 TempSet", "Head4 TempSet", "Head5 TempSet", "Head6 TempSet": Key Down {
            n143 = event-data() -> ("CtlRef"=w387:refnum<vi>, "VKey"=w383:T79)  [unwired: 1 in, 8 out]
            n144 = case shown="Default" w383 {
              tunnel: w387 -> [_ w397]
              tunnel: w386 -> [w392 w395]
              tunnel: [_ w403] -> w385
              tunnel: [w392 w394] -> w384
              frame Default {
              }
              frame "Return" {
                n145 = property class="DigNum (strict)"(reference=w397, error in=w395, "Key Focus"=FALSE, "Key Focus"=TRUE) -> (error out=w394:errorcluster, "Value"=w393:dbl, "Label.Text"=w396:string)  [unwired: 1 out]
                n146 = case shown="Default" w396 {
                  tunnel: [0.0 ("Head6 TempSet") w406 w408 w410 w412 w414 w416] -> w401
                  tunnel: [PrinterHeads--Enum."-1" ("Head") PrinterHeads--Enum."1" ("Head") PrinterHeads--Enum."2" ("Head") PrinterHeads--Enum."3" ("Head") PrinterHeads--Enum."4" ("Head") PrinterHeads--Enum."5" ("Head") PrinterHeads--Enum."6" ("Head")] -> w402
                  tunnel: w393 -> [_ w406 w408 w410 w412 w414 w416]
                  frame Default {
                  }
                  frame "Head1 TempSet" {
                  }
                  frame "Head2 TempSet" {
                  }
                  frame "Head3 TempSet" {
                  }
                  frame "Head4 TempSet" {
                  }
                  frame "Head5 TempSet" {
                  }
                  frame "Head6 TempSet" {
                  }
                }
                n147 = Format Into String(format string="Set Head Temperature>>%d>>%f", w402, w401) -> (resulting string=w403:string)  [unwired: 2 in, 1 out]
              }
            }
            n148 = call <vilib>:"Add State(s) to Queue__JKI_lib_State_Machine.vi"("State(s) in Front (\"\")"=w385, "State(s) in (\"\")"=w391) -> ("States Out"=w390:string)  [unwired: 13 in]
          }
          event "Head1 TempSet", "Head2 TempSet", "Head3 TempSet", "Head4 TempSet", "Head5 TempSet", "Head6 TempSet": Value Change {
            n149 = event-data() -> ("CtlRef"=w418:refnum<vi>, "NewVal"=w419:dbl)  [unwired: 1 in, 4 out]
            n150 = disable-structure shown="Enabled" {
              disable-tunnel: [w431 _] -> w420
              disable-tunnel: w419 -> [w429 _]
              disable-tunnel: w418 -> [w428 _]
              frame Disabled {
                n151 = property class="DigNum (strict)"(reference=w428) -> ("Label.Text"=w427:string)  [unwired: 1 in, 2 out]
                n152 = case shown="\"Head6 TempSet\"" w427 {
                  tunnel: [PrinterHeads--Enum."-1" ("Head") PrinterHeads--Enum."1" ("Head") PrinterHeads--Enum."2" ("Head") PrinterHeads--Enum."3" ("Head") PrinterHeads--Enum."4" ("Head") PrinterHeads--Enum."5" ("Head") PrinterHeads--Enum."6" ("Head")] -> w426
                  frame Default {
                    (unwired) 0.0 ("Head6 TempSet")
                  }
                  frame "Head1 TempSet" {
                  }
                  frame "Head2 TempSet" {
                  }
                  frame "Head3 TempSet" {
                  }
                  frame "Head4 TempSet" {
                  }
                  frame "Head5 TempSet" {
                  }
                  frame "Head6 TempSet" {
                  }
                }
                n153 = Format Into String(format string="Set Head Temperature>>%d>>%f" ("State(s) in Front (\"\")"), w426, w429) -> (resulting string=w431:string)  [unwired: 2 in, 1 out]
              }
              frame Enabled {
              }
            }
            n154 = call <vilib>:"Add State(s) to Queue__JKI_lib_State_Machine.vi"("State(s) in Front (\"\")"=w420, "State(s) in (\"\")"=w421) -> ("States Out"=w422:string)  [unwired: 13 in]
          }
          event Value Change {
            n155 = event-data() -> ()  [unwired: 1 in, 6 out]
            n156 = call <vilib>:"Add State(s) to Queue__JKI_lib_State_Machine.vi"("State(s) in Front (\"\")"="UI: Update Image Resolution" ("State(s) in Front (\"\")"), "State(s) in (\"\")"=w444) -> ("States Out"=w443:string)  [unwired: 13 in]
          }
          event "Settings", "Stage Control", "IPLC Process", "Drop Watch", "Printhead Service": Value Change {
            n157 = event-data() -> ("CtlRef"=w452:refnum<vi>)  [unwired: 1 in, 5 out]
            n158 = property class="Bool (strict)"(reference=w452) -> ("Label.Text"=w451:string)  [unwired: 1 in, 2 out]
            n159 = case shown="\"Drop Watch\"" w451 {
              tunnel: [MainTabs--tabs."Settings" ("Tab Control") MainTabs--tabs."Settings" ("Tab Control") MainTabs--tabs."Stage Control" ("Tab Control") MainTabs--tabs."Printer" ("Tab Control") MainTabs--tabs."Print Head Services" ("Tab Control")] -> w450
              tunnel: [w458 w461 w464 w467 w471] -> w449
              tunnel: [w458 w461 w464 w468 w470] -> w448
              tunnel: [w458 w461 w464 w467 w470] -> w447
              tunnel: [w459 w462 w464 w467 w470] -> w446
              tunnel: [w458 w461 w465 w467 w470] -> w445
              frame "Settings", Default {
                w459 = TRUE
                n160 = Not(x=w459) -> (.not. x?=w458:bool)
              }
              frame "Drop Watch" {
                w462 = TRUE
                n161 = Not(x=w462) -> (.not. x?=w461:bool)
              }
              frame "Stage Control" {
                w465 = TRUE
                n162 = Not(x=w465) -> (.not. x?=w464:bool)
              }
              frame "IPLC Process" {
                w468 = TRUE
                n163 = Not(x=w468) -> (.not. x?=w467:bool)
              }
              frame "Printhead Service" {
                w471 = TRUE
                n164 = Not(x=w471) -> (.not. x?=w470:bool)
              }
            }
            n165 = local write "Tab Control"(w450) -> ()
            n166 = local write "IPLC Process"(w448) -> ()
            n167 = local write "Drop Watch"(w447) -> ()
            n168 = local write "Settings"(w446) -> ()
            n169 = local write "Stage Control"(w445) -> ()
            n170 = local write "Printhead Service"(w449) -> ()
            n171 = call <vilib>:"Add State(s) to Queue__JKI_lib_State_Machine.vi"("State(s) in (\"\")"=w457) -> ("States Out"=w456:string)  [unwired: 14 in]
          }
          event "Analog IO": Value Change {
            n172 = event-data() -> ()  [unwired: 1 in, 6 out]
            n173 = local write "SettingsTabs"(SettinsgTabs--Tab."Analog IO" ("SettingsTabs")) -> ()
            n174 = call <vilib>:"Add State(s) to Queue__JKI_lib_State_Machine.vi"("State(s) in (\"\")"=w478) -> ("States Out"=w477:string)  [unwired: 14 in]
          }
          event "Digital IO": Value Change {
            n175 = event-data() -> ()  [unwired: 1 in, 6 out]
            n176 = local write "SettingsTabs"(SettinsgTabs--Tab."Digital IO" ("SettingsTabs")) -> ()
            n177 = call <vilib>:"Add State(s) to Queue__JKI_lib_State_Machine.vi"("State(s) in (\"\")"=w484) -> ("States Out"=w483:string)  [unwired: 14 in]
          }
          event "Script CMD": Value Change {
            n178 = event-data() -> ()  [unwired: 1 in, 6 out]
            n179 = local write "SettingsTabs"(SettinsgTabs--Tab."Script CMD" ("SettingsTabs")) -> ()
            n180 = call <vilib>:"Add State(s) to Queue__JKI_lib_State_Machine.vi"("State(s) in (\"\")"=w490) -> ("States Out"=w489:string)  [unwired: 14 in]
          }
          event "General": Value Change {
            n181 = event-data() -> ()  [unwired: 1 in, 6 out]
            n182 = local write "SettingsTabs"(SettinsgTabs--Tab."General" ("SettingsTabs")) -> ()
            n183 = call <vilib>:"Add State(s) to Queue__JKI_lib_State_Machine.vi"("State(s) in (\"\")"=w496) -> ("States Out"=w495:string)  [unwired: 14 in]
          }
          event "Load Customer Design": Value Change {
            n184 = event-data() -> ()  [unwired: 1 in, 6 out]
            n185 = property on="Recipe" class="Ring (strict)"() -> ("RingText.Text"=w503:string)  [unwired: 2 in, 2 out]
            n186 = Concatenate Strings("Data: LoadRecipe>>" ("string"), w503) -> (w500:string)
            n187 = Format Into String(format string="%s\nUI: Verify and Apply Recipe Details", error in=w497, w500) -> (resulting string=w499:string, error out=w498:errorcluster)  [unwired: 1 in]
            n188 = call <vilib>:"Add State(s) to Queue__JKI_lib_State_Machine.vi"("State(s) in Front (\"\")"=w499, "State(s) in (\"\")"=w507) -> ("States Out"=w506:string)  [unwired: 13 in]
          }
          event "AdvPrinterTabsBtn": Value Change {
            n189 = event-data() -> ("NewVal"=w511:bool)  [unwired: 1 in, 5 out]
            n190 = Select(t=AdvPrinterControl--Tabs."Adv Printer Controls" ("PrinterControls"), s=w511, f=AdvPrinterControl--Tabs."Images" ("PrinterControls")) -> (s? t:f=w508:T5)
            n191 = property on="PrinterControls" class="TabCtl (strict)"("Value"=w508) -> ()  [unwired: 2 in, 2 out]
            n192 = call <vilib>:"Add State(s) to Queue__JKI_lib_State_Machine.vi"("State(s) in (\"\")"=w516) -> ("States Out"=w515:string)  [unwired: 14 in]
          }
          event "INITIALIZATION FILE PATH", "PRODUCT RECIPE XML FOLDER PATH": Value Change {
            n193 = event-data() -> ("CtlRef"=w531:refnum<vi>, "NewVal"=w529:path)  [unwired: 1 in, 4 out]
            n194 = Unbundle By Name(w525) -> ("DLP2ConfigLoaded"=w528:T35)
            n195 = call <userlib>:"Application Directory__ogtk.vi"() -> ("Application Directory (+ Relative)"=w520:path)  [unwired: 1 in]
            n196 = property class="Path"(reference=w531) -> ("Label.Text"=w530:string)  [unwired: 1 in, 2 out]
            n197 = Build Path(base path=w520, name or relative path="startup.ini") -> (appended path=w519:path)
            n198 = case shown="\"CALIBRATION RECIPE XML FOLDER PATH\"" w530 {
              tunnel: w525 -> [w536 w549 w562 w575 w579 w583 w587 w591 w595 w599 w603 w607]
              tunnel: [w536 w549 w562 w575 w578 w582 w586 w590 w594 w598 w602 w606] -> w524
              tunnel: w529 -> [_ w541 w554 w567 w577 w581 w585 w589 w593 w597 w601 w605]
              tunnel: w519 -> [_ w548 w561 w574 _ _ _ _ _ _ _ _]
              tunnel: w517 -> [w535 w545 w558 w571 w576 w580 w584 w588 w592 w596 w600 w604]
              tunnel: [w535 w537 w550 w563 w576 w580 w584 w588 w592 w596 w600 w604] -> w518
              frame Default {
              }
              frame "INITIALIZATION FILE PATH" {
                n199 = call <vilib>:"Open Config Data.vi"("error in (no error)"=w545, "create file if necessary (T)"=FALSE, "configuration file path"=w548) -> ("error out"=w544:errorcluster, "refnum"=w547:T80)  [unwired: 6 in, 1 out]
                n200 = call-poly <vilib>:"Write Key.vi"("section"="Startup INI", "error in (no error)"=w544, "value"=w541, "key"="DLP2InitializationFilePath", "refnum"=w547) -> ("error out"=w540:errorcluster, "found?"=w539:bool, "refnum out"=w538:T80)  [unwired: 4 in]
                n201 = call <vilib>:"Close Config Data.vi"("error in (no error)"=w540, "write file if changed (T)"=w539, "refnum"=w538) -> ("error out"=w537:errorcluster)  [unwired: 7 in, 1 out]
              }
              frame "PRODUCT RECIPE XML FOLDER PATH" {
                n202 = call <vilib>:"Open Config Data.vi"("error in (no error)"=w558, "create file if necessary (T)"=FALSE, "configuration file path"=w561) -> ("error out"=w557:errorcluster, "refnum"=w560:T80)  [unwired: 6 in, 1 out]
                n203 = call-poly <vilib>:"Write Key.vi"("section"="Startup INI", "error in (no error)"=w557, "value"=w554, "key"="RecipeXMLFolder", "refnum"=w560) -> ("error out"=w553:errorcluster, "found?"=w552:bool, "refnum out"=w551:T80)  [unwired: 4 in]
                n204 = call <vilib>:"Close Config Data.vi"("error in (no error)"=w553, "write file if changed (T)"=w552, "refnum"=w551) -> ("error out"=w550:errorcluster)  [unwired: 7 in, 1 out]
              }
              frame "CALIBRATION RECIPE XML FOLDER PATH" {
                n205 = call <vilib>:"Open Config Data.vi"("error in (no error)"=w571, "create file if necessary (T)"=FALSE, "configuration file path"=w574) -> ("error out"=w570:errorcluster, "refnum"=w573:T80)  [unwired: 6 in, 1 out]
                n206 = call-poly <vilib>:"Write Key.vi"("section"="Startup INI", "error in (no error)"=w570, "value"=w567, "key"="CalibrationRecipeXMLFolder", "refnum"=w573) -> ("error out"=w566:errorcluster, "found?"=w565:bool, "refnum out"=w564:T80)  [unwired: 4 in]
                n207 = call <vilib>:"Close Config Data.vi"("error in (no error)"=w566, "write file if changed (T)"=w565, "refnum"=w564) -> ("error out"=w563:errorcluster)  [unwired: 7 in, 1 out]
              }
              frame "DigiBit WG Design Folder" {
                n208 = Bundle By Name(cluster=w579, "DLP2Config.Paths.DigiBit WG Design Folder"=w577) -> (w578:T77)
              }
              frame "Compensated GS Image Folder" {
                n209 = Bundle By Name(cluster=w583, "DLP2Config.Paths.Compensated GS Image Folder"=w581) -> (w582:T77)
              }
              frame "Head 1" {
                n210 = Bundle By Name(cluster=w587, "DLP2Config.Paths.Nozzle GS Files Head 1"=w585) -> (w586:T77)
              }
              frame "Head 2" {
                n211 = Bundle By Name(cluster=w591, "DLP2Config.Paths.Nozzle GS Files Head 2"=w589) -> (w590:T77)
              }
              frame "Head 3" {
                n212 = Bundle By Name(cluster=w595, "DLP2Config.Paths.Nozzle GS Files Head 3"=w593) -> (w594:T77)
              }
              frame "Head 4" {
                n213 = Bundle By Name(cluster=w599, "DLP2Config.Paths.Nozzle GS Files Head 4"=w597) -> (w598:T77)
              }
              frame "Head 5" {
                n214 = Bundle By Name(cluster=w603, "DLP2Config.Paths.Nozzle GS Files Head 5"=w601) -> (w602:T77)
              }
              frame "Head 6" {
                n215 = Bundle By Name(cluster=w607, "DLP2Config.Paths.Nozzle GS Files Head 6"=w605) -> (w606:T77)
              }
            }
            n216 = Unbundle By Name(w524) -> ("DLP2Config"=w527:T35)
            n217 = Not Equal?(x=w528, y=w527) -> (x != y?=w526:bool)
            n218 = Bundle By Name(cluster=w524, "ConfigSaveRequired"=w526) -> (w523:T77)
            n219 = call <vilib>:"Add State(s) to Queue__JKI_lib_State_Machine.vi"("State(s) in Front (\"\")"="UI: CheckConfigRequired" ("State(s) in Front (\"\")"), "State(s) in (\"\")"=w534) -> ("States Out"=w533:string)  [unwired: 13 in]
          }
          event "Head 1 Material", "Head 2 Material", "Head 3 Material", "Head 4 Material", "Head 5 Material", "Head 6 Material", "Head 1 ColorPlane", "Head 2 ColorPlane", "Head 3 ColorPlane", "Head 4 ColorPlane", "Head 5 ColorPlane", "Head 6 ColorPlane": Value Change {
            n220 = event-data() -> ("CtlRef"=w617:refnum<vi>)  [unwired: 1 in, 5 out]
            n221 = property class="Ring (strict)"(reference=w617) -> ("Label.Text"=w616:string, "RingText.Text"=w615:string)  [unwired: 1 in, 2 out]
            n222 = Unbundle By Name(w611) -> ("DLP2ConfigLoaded"=w610:T35)
            n223 = case shown="\"Head 1 ColorPlane\"" w616 {
              tunnel: w611 -> [w622 w625 w628 w631 w634 w637 w640 w643 w646 w649 w652 w655 w658]
              tunnel: [w622 w624 w627 w630 w633 w636 w639 w642 w645 w648 w651 w654 w657] -> w613
              tunnel: w615 -> [_ w623 w626 w629 w632 w635 w638 w641 w644 w647 w650 w653 w656]
              frame Default {
              }
              frame "Head 1 Material" {
                n224 = Bundle By Name(cluster=w625, "DLP2Config.ColorPaneMapping.Head 1.Material"=w623) -> (w624:T77)
              }
              frame "Head 1 ColorPlane" {
                n225 = Bundle By Name(cluster=w628, "DLP2Config.ColorPaneMapping.Head 1.ColorPane"=w626) -> (w627:T77)
              }
              frame "Head 2 Material" {
                n226 = Bundle By Name(cluster=w631, "DLP2Config.ColorPaneMapping.Head 1.Material"=w629) -> (w630:T77)
              }
              frame "Head 2 ColorPlane" {
                n227 = Bundle By Name(cluster=w634, "DLP2Config.ColorPaneMapping.Head 1.ColorPane"=w632) -> (w633:T77)
              }
              frame "Head 3 Material" {
                n228 = Bundle By Name(cluster=w637, "DLP2Config.ColorPaneMapping.Head 1.Material"=w635) -> (w636:T77)
              }
              frame "Head 3 ColorPlane" {
                n229 = Bundle By Name(cluster=w640, "DLP2Config.ColorPaneMapping.Head 1.ColorPane"=w638) -> (w639:T77)
              }
              frame "Head 4 Material" {
                n230 = Bundle By Name(cluster=w643, "DLP2Config.ColorPaneMapping.Head 1.Material"=w641) -> (w642:T77)
              }
              frame "Head 4 ColorPlane" {
                n231 = Bundle By Name(cluster=w646, "DLP2Config.ColorPaneMapping.Head 1.ColorPane"=w644) -> (w645:T77)
              }
              frame "Head 5 Material" {
                n232 = Bundle By Name(cluster=w649, "DLP2Config.ColorPaneMapping.Head 1.Material"=w647) -> (w648:T77)
              }
              frame "Head 5 ColorPlane" {
                n233 = Bundle By Name(cluster=w652, "DLP2Config.ColorPaneMapping.Head 1.ColorPane"=w650) -> (w651:T77)
              }
              frame "Head 6 Material" {
                n234 = Bundle By Name(cluster=w655, "DLP2Config.ColorPaneMapping.Head 1.Material"=w653) -> (w654:T77)
              }
              frame "Head 6 ColorPlane" {
                n235 = Bundle By Name(cluster=w658, "DLP2Config.ColorPaneMapping.Head 1.ColorPane"=w656) -> (w657:T77)
              }
            }
            n236 = Unbundle By Name(w613) -> ("DLP2Config"=w609:T35)
            n237 = Not Equal?(x=w610, y=w609) -> (x != y?=w608:bool)
            n238 = Bundle By Name(cluster=w613, "ConfigSaveRequired"=w608) -> (w612:T77)
